vi "open_python_test.vi"() -> ()   [LabVIEW 2022 SP3]
panel:
  in  "图片/视频路径":string
  in  "use_gpu":i32
  out "Python程序路径 2":path
  out "error out":errorcluster
  out "return value":i32
  out "错误输出":errorcluster
  out "返回值":i32
  out "Python程序路径":path
  in  "mode":i32
  in  "timeF":i32
  in  "a":dbl
  in  "b":dbl
  out "返回值 2":dbl
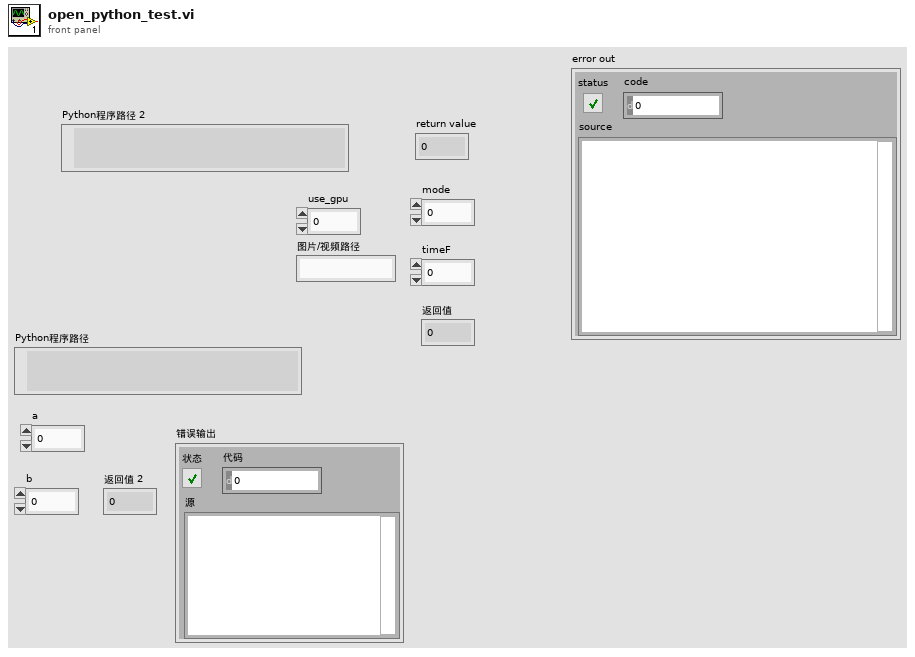
[diagram p1: front panel]
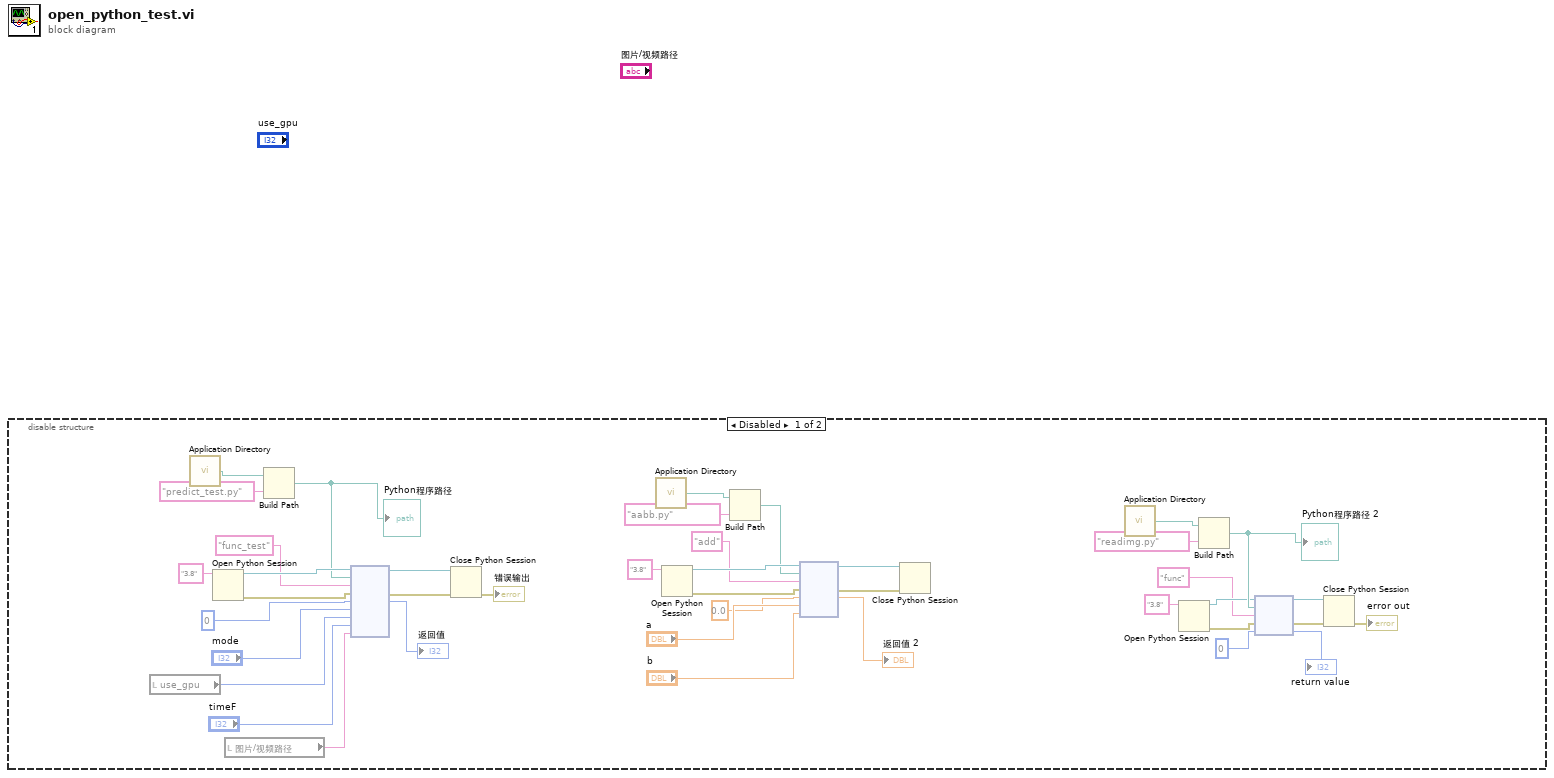
[diagram p0: block diagram]
diagram:
  n1 = disable-structure shown="Disabled" {
    frame Disabled {
      n2 = local read "use_gpu"() -> (w14:i32)
      n3 = call <vilib>:"Application Directory.vi"() -> ("Application Directory"=w29:path)
      n4 = Open Python Session(python version="3.8" ("Python版本")) -> (session out=w28:refnum<k35>, error out=w25:errorcluster)  [unwired: 2 in]
      n5 = local read "图片/视频路径"() -> (w15:string)
      n6 = Build Path(base path=w29, name or relative path="predict_test.py" ("名称或相对路径")) -> (appended path=w22:path)
      "Python程序路径" <- w22
      n7 = node(w28, w22, "func_test" ("函数名称"), w25, 0, "mode", w14, "timeF", w15) -> (w27:refnum<k35>, w26:errorcluster, →"返回值":i32)  [unwired: 4 in, 2 out]
      n8 = Close Python Session(session in=w27, error in=w26) -> (11:→"错误输出":errorcluster)
      n9 = call <vilib>:"Application Directory.vi"() -> ("Application Directory"=w12:path)
      n10 = Open Python Session(python version="3.8" ("Python版本")) -> (session out=w13:refnum<k35>, error out=w8:errorcluster)  [unwired: 2 in]
      n11 = Build Path(base path=w12, name or relative path="aabb.py" ("名称或相对路径")) -> (appended path=w11:path)
      n12 = node(w13, w11, "add" ("函数名称"), w8, 0.0, "a", "b") -> (w10:refnum<k35>, w9:errorcluster, →"返回值 2":dbl)  [unwired: 2 in, 2 out]
      n13 = Close Python Session(session in=w10, error in=w9) -> ()  [unwired: 1 out]
      n14 = call <vilib>:"Application Directory.vi"() -> ("Application Directory"=w35:path)
      n15 = Open Python Session(python version="3.8" ("Python版本")) -> (session out=w34:refnum<k35>, error out=w37:errorcluster)  [unwired: 2 in]
      n16 = Build Path(base path=w35, name or relative path="readimg.py" ("名称或相对路径")) -> (appended path=w36:path)
      "Python程序路径 2" <- w36
      n17 = node(w34, w36, "func" ("函数名称"), w37, 0) -> (w38:refnum<k35>, w39:errorcluster, →"return value":i32)  [unwired: 2 out]
      n18 = Close Python Session(session in=w38, error in=w39) -> (11:→"error out":errorcluster)
    }
    frame Enabled {
    }
  }
